vi "Sequences_of_Elements_Retrieved.vi"(8 "Element3":variant, 9 "Element2":variant, 10 "Element1":variant, 11 "Array_Retrieved":variant[][](array[variant])) -> (2 "All_Data_Sequences":i32[](array[numeric]))   [LabVIEW 2019]
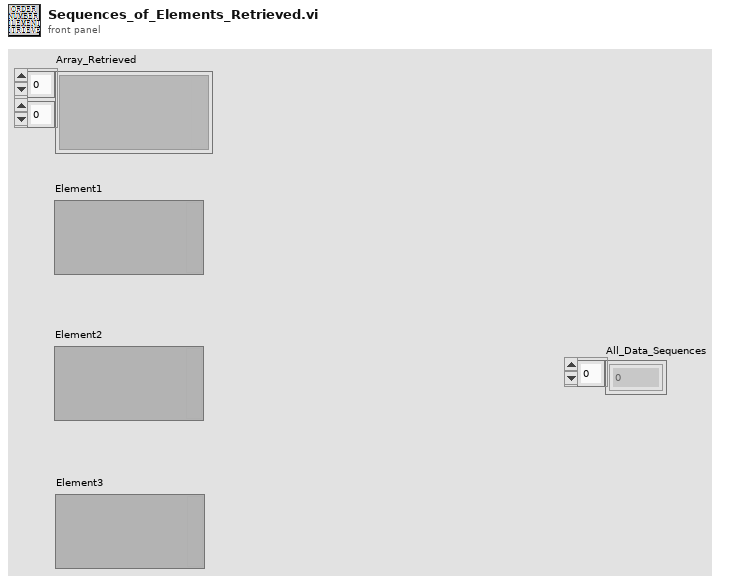
[diagram p1: front panel]
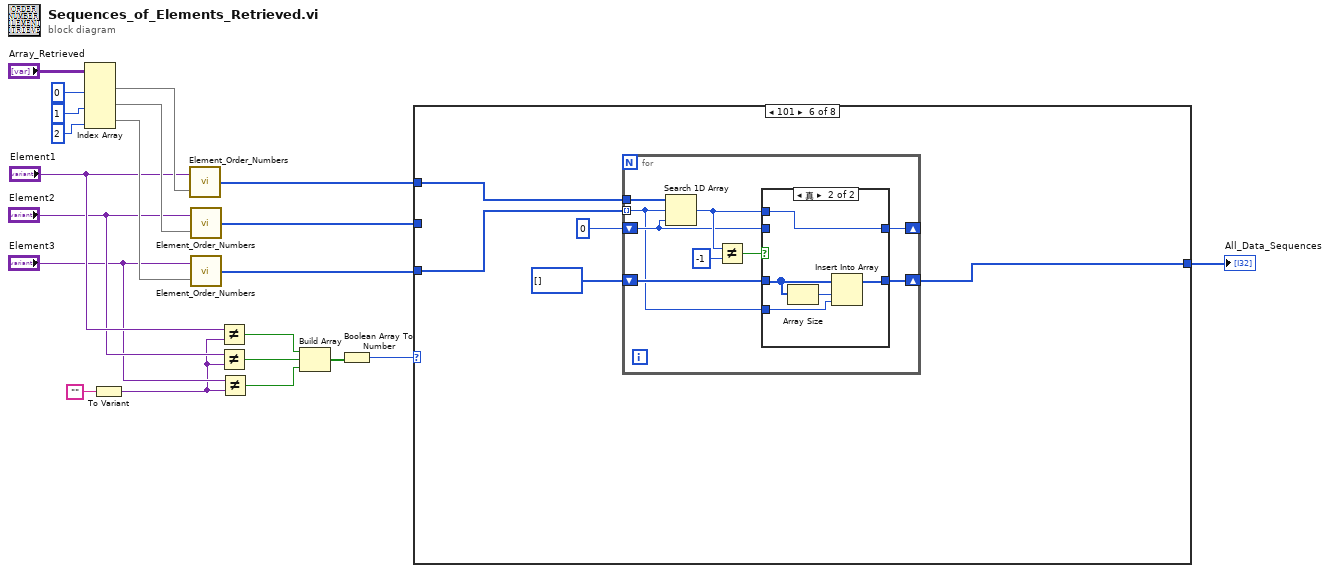
[diagram p0: block diagram]
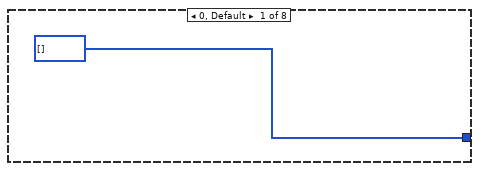
[diagram p2: hidden frame]
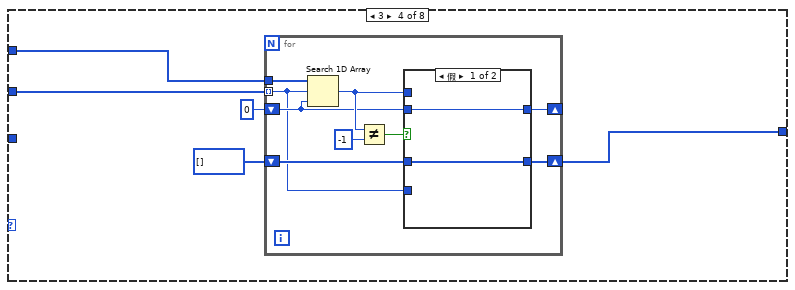
[diagram p5: hidden frame]
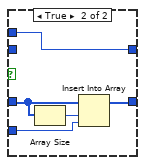
[diagram p6: hidden frame]
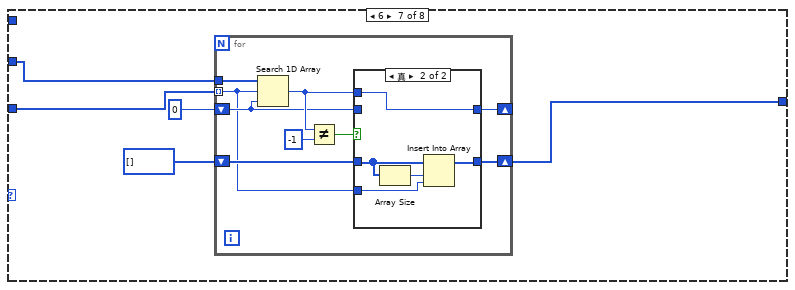
[diagram p9: hidden frame]
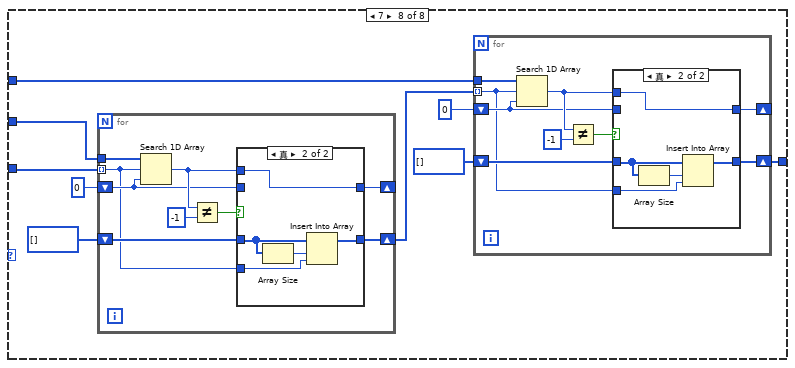
[diagram p11: hidden frame]
diagram:
  n1 = Index Array(array="Array_Retrieved", index (col) #1=0, index (col) #2=1, index (col) #3=2) -> (element #1=w17:variant[], element #2=w16:variant[], element #3=w15:variant[])  [unwired: 3 in]
  n2 = To Variant(anything="") -> (Variant=w1:variant)
  n3 = call "Element_Order_Numbers.vi"("Element_Array"=w17, "Element"="Element1") -> ("Order_numbers"=w13:i32[])
  n4 = call "Element_Order_Numbers.vi"("Element_Array"=w16, "Element"="Element2") -> ("Order_numbers"=w12:i32[])
  n5 = call "Element_Order_Numbers.vi"("Element_Array"=w15, "Element"="Element3") -> ("Order_numbers"=w11:i32[])
  n6 = Not Equal?(x="Element1", y=w1) -> (x != y?=w6:bool)
  n7 = Not Equal?(x="Element2", y=w1) -> (x != y?=w5:bool)
  n8 = Not Equal?(x="Element3", y=w1) -> (x != y?=w4:bool)
  n9 = Build Array(w6, w5, w4) -> (w3:bool[])
  n10 = Boolean Array To Number(Boolean array=w3) -> (number=w14:u32)
  n11 = case shown="101" w14 {
    tunnel: [i32[] [] w23 w24 w25 w46 w47 w68 w90] -> w10
    tunnel: w13 -> [_ w23 _ w27 _ w49 _ w91]
    tunnel: w12 -> [_ _ w24 w26 _ _ w70 w95]
    tunnel: w11 -> [_ _ _ _ w46 w48 w69 w94]
    frame 0, Default {
    }
    frame 1 {
    }
    frame 2 {
    }
    frame 3 {
      n12 = for {
        tunnel: w27 -> [w38]
        tunnel: w26 -> [w30] mode=indexing
        shift-right: [w35] -> _
        shift-left: 0 -> [w31]
        shift-right: [w33] -> w25
        shift-left: i32[] [] -> [w34]
        n13 = Search 1D Array(1D array=w38, element=w30, start index (0)=w31) -> (index of element=w32:i32)
        n14 = Not Equal?(x=w32, y=-1) -> (x != y?=w36:bool)
        n15 = case shown="假" w36 {
          tunnel: [w40 w42] -> w35
          tunnel: w31 -> [w40 _]
          tunnel: w34 -> [w39 w43]
          tunnel: [w39 w44] -> w33
          tunnel: w32 -> [_ w42]
          tunnel: w30 -> [_ w41]
          frame False {
          }
          frame True {
            n16 = Array Size(array=w43) -> (size(s)=w45:i32)
            n17 = Insert Into Array(array=w43, index=w45, new element=w41) -> (w44:i32[])
          }
        }
      }
    }
    frame 4 {
    }
    frame 5 {
      n18 = for {
        tunnel: w49 -> [w60]
        tunnel: w48 -> [w52] mode=indexing
        shift-right: [w57] -> _
        shift-left: 0 -> [w53]
        shift-right: [w55] -> w47
        shift-left: i32[] [] -> [w56]
        n19 = Search 1D Array(1D array=w60, element=w52, start index (0)=w53) -> (index of element=w54:i32)
        n20 = Not Equal?(x=w54, y=-1) -> (x != y?=w58:bool)
        n21 = case shown="真" w58 {
          tunnel: [w62 w64] -> w57
          tunnel: w53 -> [w62 _]
          tunnel: w56 -> [w61 w65]
          tunnel: [w61 w66] -> w55
          tunnel: w54 -> [_ w64]
          tunnel: w52 -> [_ w63]
          frame False {
          }
          frame True {
            n22 = Array Size(array=w65) -> (size(s)=w67:i32)
            n23 = Insert Into Array(array=w65, index=w67, new element=w63) -> (w66:i32[])
          }
        }
      }
    }
    frame 6 {
      n24 = for {
        tunnel: w70 -> [w81]
        tunnel: w69 -> [w73] mode=indexing
        shift-right: [w78] -> _
        shift-left: 0 -> [w74]
        shift-right: [w76] -> w68
        shift-left: i32[] [] -> [w77]
        n25 = Search 1D Array(1D array=w81, element=w73, start index (0)=w74) -> (index of element=w75:i32)
        n26 = Not Equal?(x=w75, y=-1) -> (x != y?=w79:bool)
        n27 = case shown="真" w79 {
          tunnel: [w83 w85] -> w78
          tunnel: w74 -> [w83 _]
          tunnel: w77 -> [w82 w86]
          tunnel: [w82 w87] -> w76
          tunnel: w75 -> [_ w85]
          tunnel: w73 -> [_ w84]
          frame False {
          }
          frame True {
            n28 = Array Size(array=w86) -> (size(s)=w88:i32)
            n29 = Insert Into Array(array=w86, index=w88, new element=w84) -> (w87:i32[])
          }
        }
      }
    }
    frame 7 {
      n30 = for {
        tunnel: w95 -> [w122]
        tunnel: w94 -> [w114] mode=indexing
        shift-right: [w119] -> _
        shift-left: 0 -> [w115]
        shift-right: [w117] -> w92
        shift-left: i32[] [] -> [w118]
        n31 = Search 1D Array(1D array=w122, element=w114, start index (0)=w115) -> (index of element=w116:i32)
        n32 = Not Equal?(x=w116, y=-1) -> (x != y?=w120:bool)
        n33 = case shown="真" w120 {
          tunnel: [w124 w126] -> w119
          tunnel: w115 -> [w124 _]
          tunnel: w118 -> [w123 w127]
          tunnel: [w123 w128] -> w117
          tunnel: w116 -> [_ w126]
          tunnel: w114 -> [_ w125]
          frame False {
          }
          frame True {
            n34 = Array Size(array=w127) -> (size(s)=w129:i32)
            n35 = Insert Into Array(array=w127, index=w129, new element=w125) -> (w128:i32[])
          }
        }
      }
      n36 = for {
        tunnel: w91 -> [w106]
        tunnel: w92 -> [w98] mode=indexing
        shift-right: [w103] -> _
        shift-left: 0 -> [w99]
        shift-right: [w101] -> w90
        shift-left: i32[] [] -> [w102]
        n37 = Search 1D Array(1D array=w106, element=w98, start index (0)=w99) -> (index of element=w100:i32)
        n38 = Not Equal?(x=w100, y=-1) -> (x != y?=w104:bool)
        n39 = case shown="真" w104 {
          tunnel: [w108 w110] -> w103
          tunnel: w99 -> [w108 _]
          tunnel: w102 -> [w107 w111]
          tunnel: [w107 w112] -> w101
          tunnel: w100 -> [_ w110]
          tunnel: w98 -> [_ w109]
          frame False {
          }
          frame True {
            n40 = Array Size(array=w111) -> (size(s)=w113:i32)
            n41 = Insert Into Array(array=w111, index=w113, new element=w109) -> (w112:i32[])
          }
        }
      }
    }
  }
  "All_Data_Sequences" <- w10
